vi "swap.vi"(8 "error in (no error)":errorcluster, 10 "target storage mode":T1, 11 "ImageCollection in":refnum<class "ImageCollection.lvclass">) -> (0 "error out":errorcluster, 3 "ImageCollection out":refnum<class "ImageCollection.lvclass">, 4 "previous storage mode":T1)   [LabVIEW 2010, in "ImageCollection.lvclass"]
uses:
  ImageCollection.lvclass
  storage_mode_enum.ctl
  Image/Image/storage_mode.ctl
  Image/Image/Image.lvclass
  ImageCollection.lvclass/ImageCollection.ctl
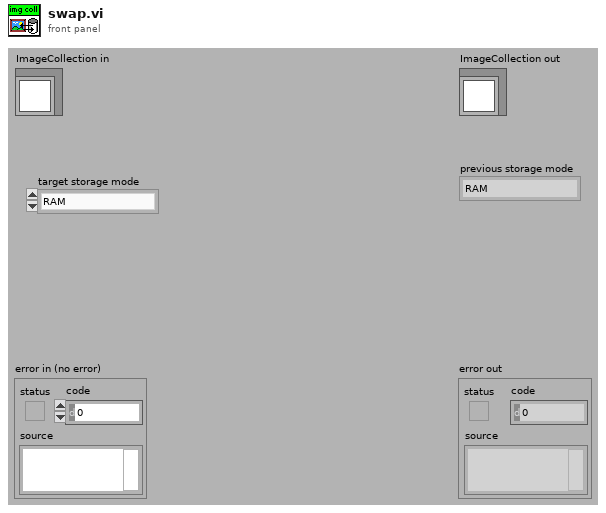
[diagram p1: front panel]
types:
  T1 = typedef "ImageCollection.lvclass/storage_mode_enum.ctl" = enum16{"RAM", "single files", "multipage TIFF (read-only)"}
  T2 = typedef "Image.lvclass/storage_mode.ctl" = enum16{"RAM", "disk"}
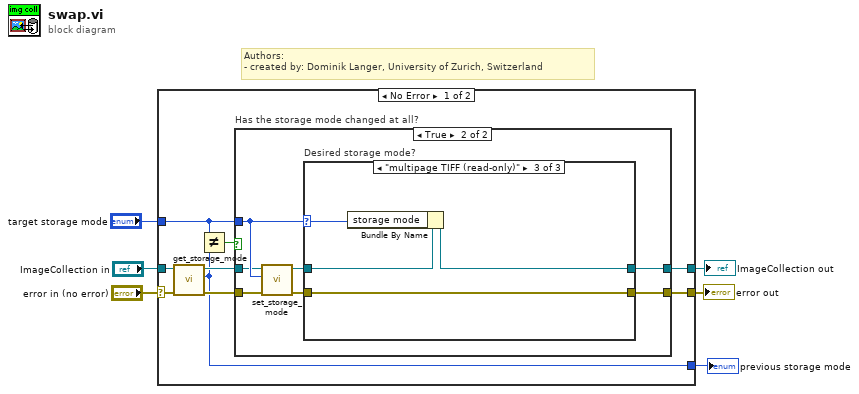
[diagram p0: block diagram]
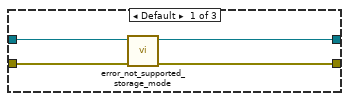
[diagram p3: hidden frame]
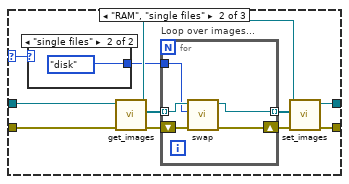
[diagram p4: hidden frame]
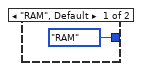
[diagram p5: hidden frame]
diagram:
  # "Authors: \n- created by: Dominik Langer, University of Zurich, Switzerland"
  n1 = case shown="No Error" "error in (no error)" {
    selector: "error in (no error)" -> [w15 w51]
    tunnel: [w9 w51] -> w3
    tunnel: [w8 w52] -> w2
    tunnel: "ImageCollection in" -> [w13 w52]
    tunnel: "target storage mode" -> [w12 _]
    tunnel: [w7 _] -> w1
    frame No Error {
      n2 = call-dynamic "get_storage_mode.vi"("error in (no error)"=w15, "ImageCollection.lvclass in"=w13) -> ("error out"=w14:errorcluster, "storage type"=w7:T1, "ImageCollection.lvclass out"=w10:refnum<class "ImageCollection.lvclass">)  [unwired: 7 out]
      n3 = Not Equal?(x=w12, y=w7) -> (x != y?=w11:bool)
      n4 = case "Has the storage mode changed at all?" shown="True" w11 {
        tunnel: w14 -> [w16 w21]
        tunnel: w10 -> [w17 w20]
        tunnel: w12 -> [_ w24]
        tunnel: [w16 w19] -> w9
        tunnel: [w17 w18] -> w8
        frame False {
        }
        frame True {
          n5 = call-dynamic "set_storage_mode.vi"("error in (no error)"=w21, "type"=w24, "ImageCollection.lvclass in"=w20) -> ("error out"=w23:errorcluster, "ImageCollection.lvclass out"=w22:refnum<class "ImageCollection.lvclass">)  [unwired: 7 out]
          n6 = case "Desired storage mode?" shown="\"multipage TIFF (read-only)\"" w24 {
            selector: w24 -> [_ w30 w47]
            tunnel: [w25 w39 w48] -> w18
            tunnel: [w26 w38 w50] -> w19
            tunnel: w23 -> [w28 w33 w50]
            tunnel: w22 -> [w27 w32 w49]
            frame Default {
              n7 = call-dynamic "error_not_supported_storage_mode.vi"("error in (no error)"=w28, "ImageCollection in"=w27) -> ("error out"=w26:errorcluster, "ImageCollection out"=w25:refnum<class "ImageCollection.lvclass">)  [unwired: 8 out]
            }
            frame "RAM", "single files" {
              n8 = case shown="\"single files\"" w30 {
                tunnel: [storage_mode."RAM" ("storage type") storage_mode."disk" ("storage type")] -> w29
                frame "RAM", Default {
                }
                frame "single files" {
                }
              }
              n9 = call-dynamic "get_images.vi"("error in (no error)"=w33, "ImageCollection.lvclass in"=w32) -> ("error out"=w36:errorcluster, "images"=w37:refnum<class "Image.lvclass">[], "ImageCollection.lvclass out"=w31:refnum<class "ImageCollection.lvclass">)  [unwired: 1 in, 6 out]
              n10 = for "Loop over images..." {
                tunnel: w37 -> [w45] mode=indexing
                tunnel: [w44] -> w35 mode=indexing
                shift-right: [w42] -> w34
                shift-left: w36 -> [w46]
                tunnel: w29 -> [w43]
                n11 = call-dynamic "swap.vi"("error in (no error)"=w46, "storage type target"=w43, "Image in"=w45) -> ("error out"=w42:errorcluster, "Image out"=w44:refnum<class "Image.lvclass">)  [unwired: 7 out]
              }
              n12 = call-dynamic "set_images.vi"("error in (no error)"=w34, "images"=w35, "ImageCollection.lvclass in"=w31) -> ("error out"=w38:errorcluster, "ImageCollection.lvclass out"=w39:refnum<class "ImageCollection.lvclass">)  [unwired: 7 out]
            }
            frame "multipage TIFF (read-only)" {
              n13 = Bundle By Name(cluster=w49, "storage mode"=w47) -> (w48:refnum<class "ImageCollection.lvclass">)
            }
          }
        }
      }
    }
    frame Error {
    }
  }
  "error out" <- w3
  "ImageCollection out" <- w2
  "previous storage mode" <- w1
